vi "D3DM_Top.vi"() -> ()   [LabVIEW 2013]
panel:
  out "graphic cluster 2":cluster{}
  out "data cluster":cluster{}
  in  "control cluster":cluster{}
  in  "config input":cluster{}
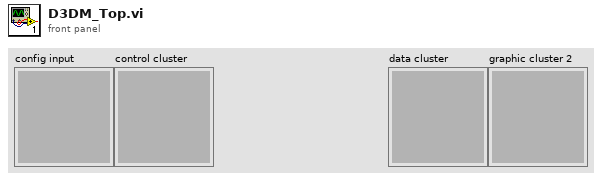
[diagram p1: front panel]
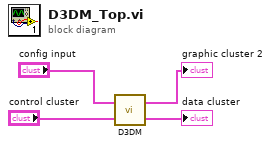
[diagram p0: block diagram]
diagram:
  n1 = call "D3DM.vi"("control cluster"="control cluster", "config input"="config input") -> ("data cluster"=→"data cluster":cluster{}, "graphic cluster"=→"graphic cluster 2":cluster{})
